vi "Folder name timestamp.vi"() -> (3 "date/time string":string)   [LabVIEW 2013]
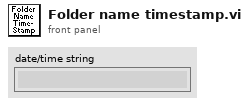
[diagram p1: front panel]
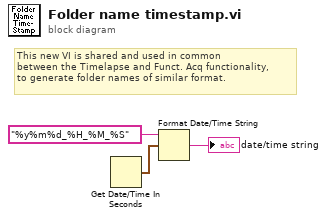
[diagram p0: block diagram]
diagram:
  # "This new VI is shared and used in common\nbetween the Timelapse and Funct. Acq functionality,\nto generate folder names of similar format."
  n1 = Get Date/Time In Seconds() -> (seconds since 1Jan1904=w2:timestamp)
  n2 = Format Date/Time String(time format string (%c)="%y%m%d_%H_%M_%S", seconds (now)=w2) -> (date/time string=→"date/time string":string)  [unwired: 1 in]
